vi "Intake Controller.vi"(8 "error in":errorcluster) -> ()   [LabVIEW 2019]
doc: "This VI executes continuously carrying out the current operation and responding to updates or new operations. It will often contain the timing or control code that is difficult to place directly in TeleOp. This VI generally opens all sensors and motors and isolates the rest of the robot code from knowing how the operations are carried out."
uses:
  <vilib>/Rock Robotics/WPI/Framework/Completion Status.ctl
  Intake Setpoints.ctl
  Intake Operations.ctl
  <vilib>/Rock Robotics/WPI/ThirdParty/Phoenix-LabVIEW/Motor Controller/Controls/CTRE_Phoenix_MotorControl_ControlMode.ctl
  <vilib>/Rock Robotics/Network Tables/NT Write Boolean.vi
panel:
  in  "Interactive Values":T1
  out "Current\nCmd":string
  in  "Buttons":cluster{"Execute Cmd":bool, "Abort Cmd":bool}
  out "Command Timing":cluster{"Start Time (ms)":u32, "Iterations":i32}
  out "Status":T3
  # "Tip: It may be helpful to observe inputs and sensor values.\nYou may also want to display tuning or debugging controls."
  # "Interactive Command: You may fill in the settings for a command\nand schedule it with the Execute button. You can observe and abort\nany command while fine tuning the code for the controller."
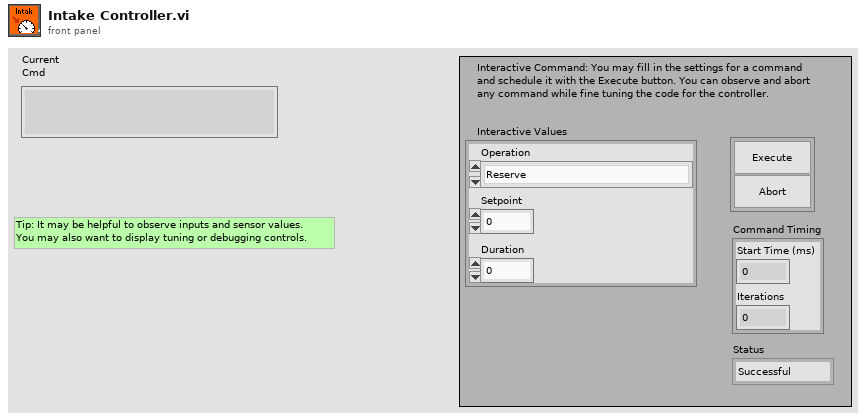
[diagram p1: front panel]
types:
  T1 = typedef "Intake Setpoints.ctl" = cluster{"Operation":T2, "Setpoint":dbl, "Duration":dbl}
  T2 = typedef "Intake Operations.ctl" = enum16{"Reserve", "Read Current", "Immediate", "Intake for time"}
  T3 = typedef "Completion Status.ctl" = enum16{"Successful", "Aborted", "Incomplete"}
  T4 = typedef "WPI_MotorControlDeviceRef.ctl" = cluster{"DeviceStatus":errorcluster, "Type":T5, "PWM":cluster{"PWM Channel":T6, "DeadBand":T7}, "CAN":cluster{"Device Number":u8, "SetOutput VI Ref":variant, "GetOutput VI Ref":variant, "Enable VI Ref":variant, "Disable VI Ref":variant, "Data":variant}, "Invert":bool, "DIO PWM":cluster{"PWM \"Enable\" Channel":T6, "DIOChannel":T8, "PWM Rate":dbl}}
  T5 = typedef "WPI_MotorControlType.ctl" = enum16{"PWM", "CAN", "DIO PWM"}
  T6 = typedef "FPGA_DIOPWMChannel.ctl" = enum8{"PWM 0", "PWM 1", "PWM 2", "PWM 3", "PWM 4", "PWM 5", "PWM 6", "PWM 7", "PWM 8", "PWM 9", "PWM MXP 0", "PWM MXP 1", "PWM MXP 2", "PWM MXP 3", "PWM MXP 4", "PWM MXP 5", "PWM MXP 6", "PWM MXP 7", "PWM MXP 8", "PWM MXP 9", "Invalid"}
  T7 = typedef "WPI_PWMDeadband.ctl" = cluster{"Name":string, "maxPositivePwm":i32, "minPositivePwm":i32, "centerPwm":i32, "maxNegativePwm":i32, "minNegativePwm":i32, "angularRange":u16}
  T8 = typedef "FPGA_DIOChannel.ctl" = enum8{"DIO 0", "DIO 1", "DIO 2", "DIO 3", "DIO 4", "DIO 5", "DIO 6", "DIO 7", "DIO 8", "DIO 9", "DIO MXP 0", "DIO MXP 1", "DIO MXP 2", "DIO MXP 3", "DIO MXP 4", "DIO MXP 5", "DIO MXP 6", "DIO MXP 7", "DIO MXP 8", "DIO MXP 9", "DIO MXP 10", "DIO MXP 11", "DIO MXP 12", "DIO MXP 13", "DIO MXP 14", "DIO MXP 15", "SPI Port CS1", "SPI Port CS2", "SPI Port CS3", "SPI Port MISO", "SPI Port MOSI", "Invalid"}
  T9 = typedef "Command Status Info.ctl" = cluster{"Name":string, "Status":T3, "notifier out":T10}
  T10 = typedef "Completion Notifier.ctl" = refnum<notifier>
  T11 = cluster{"Current Command":T1, "Command Timing":cluster{"Start Time (ms)":u32, "Iterations":i32}, "Command Arguments":cluster{"Command Info":T9, "Description":string, "Default Command":T1, "queue out":refnum<queue>, "Subsystem Name":string}}
  T12 = typedef "CTRE_Phoenix_MotorControl_ControlMode.ctl" = u16
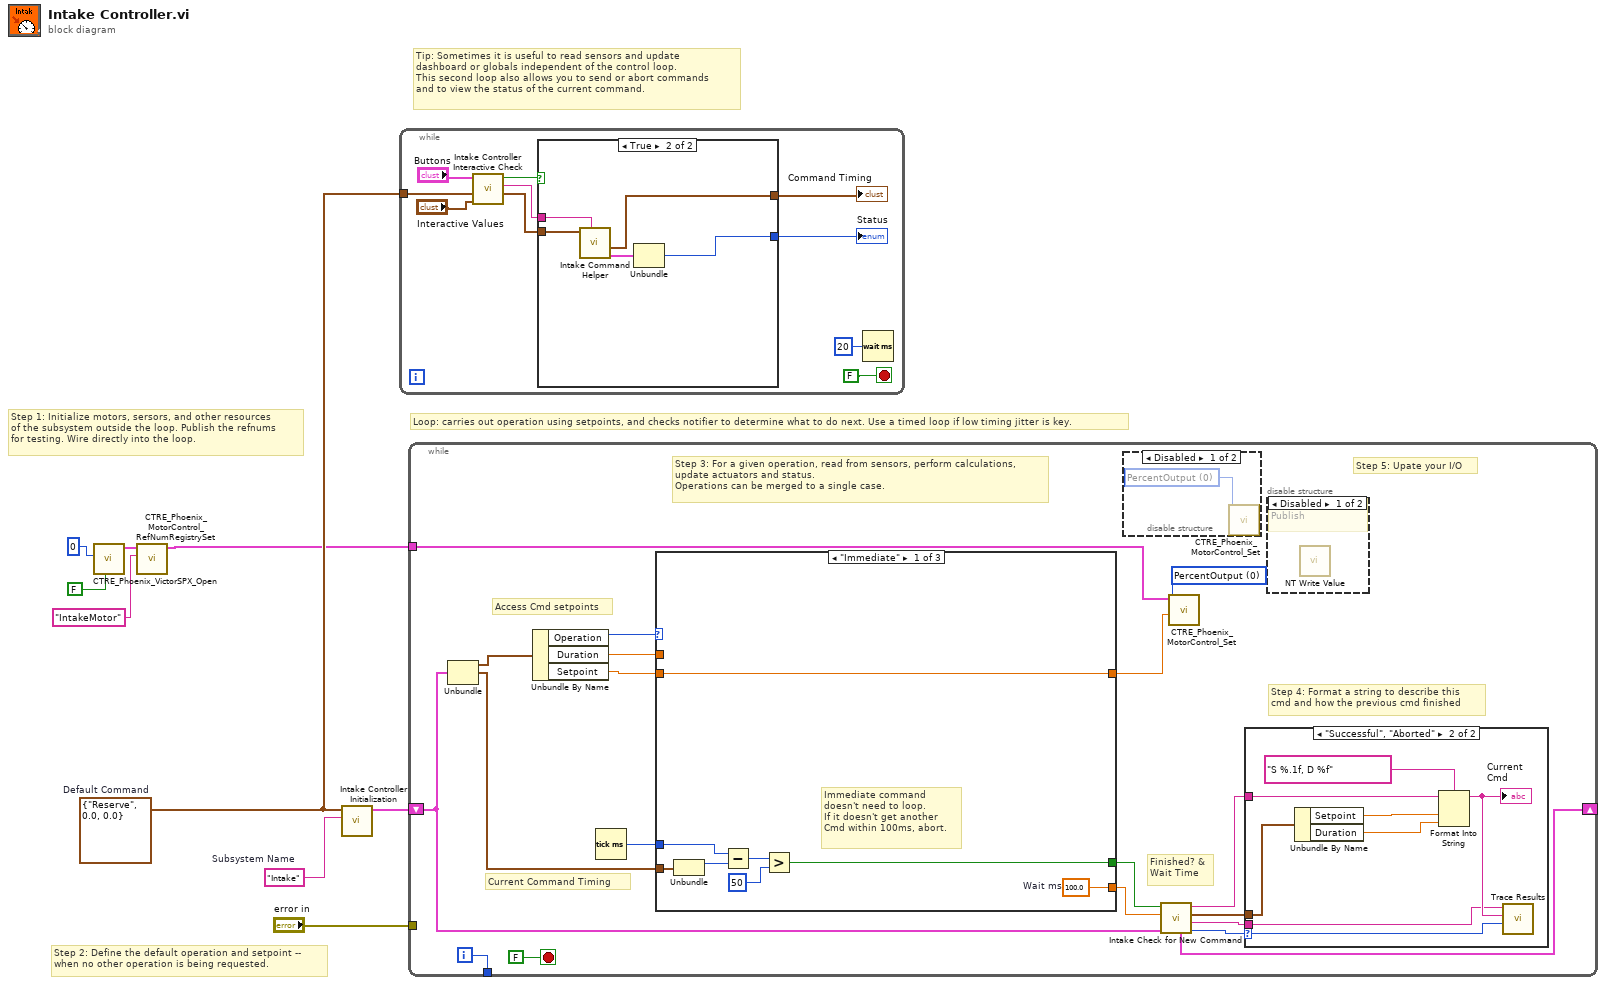
[diagram p0: block diagram]
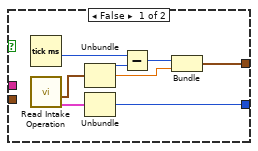
[diagram p2: hidden frame]
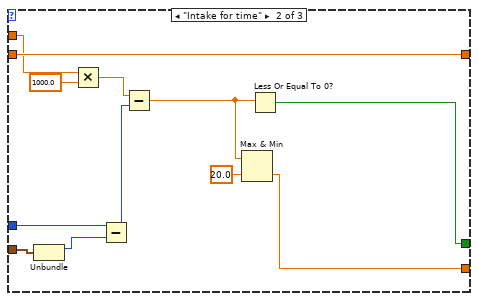
[diagram p6: hidden frame]
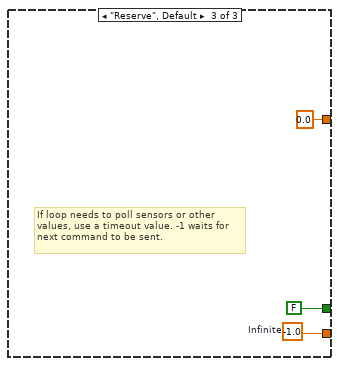
[diagram p7: hidden frame]
diagram:
  w6 = T1 {"Operation"=enum."Reserve", "Setpoint"=0.0, "Duration"=0.0}  # Default Command
  w7 = "Intake"  # Subsystem Name
  # "Tip: Sometimes it is useful to read sensors and update\ndashboard or globals independent of the control loop.\nThis second loop also allows you to send or abort commands\nand to view the status of the current command."
  # "Step 2: Define the default operation and setpoint --\nwhen no other operation is being requested."
  # "Step 1: Initialize motors, sersors, and other resources\nof the subsystem outside the loop. Publish the refnums\nfor testing. Wire directly into the loop."
  # "Loop: carries out operation using setpoints, and checks notifier to determine what to do next. Use a timed loop if low timing jitter is key."
  n1 = call <vilib>:"CTRE_Phoenix_VictorSPX_Open.vi"("Invert"=FALSE, "Device Number"=u8 0) -> ("CAN Talon SRX Ref"=w4:T4)  [unwired: 8 in, 1 out]
  n2 = call <vilib>:"CTRE_Phoenix_MotorControl_RefNumRegistrySet.vi"("refnum name"="IntakeMotor", "PhoenixMotorControlDevRef"=w4) -> ("PhoenixMotorControlDevRef"=w1:T4)  [unwired: 8 in, 1 out]
  n3 = call "Intake Controller Initialization.vi"("Subsystem Name"=w7, "Default Command"=w6) -> ("Current Command"=w8:T11)  [unwired: 9 in]
  n4 = while {
    tunnel: w6 -> [w16]
    stop <- FALSE stop-if-true
    n5 = call "Intake Controller Interactive Check.vi"("Interactive Command in"="Interactive Values", "Default Command"=w16, "Buttons"="Buttons") -> ("Interactive Command out"=w13:T1, "Trace String"=w14:string, "Schedule"=w15:bool)  [unwired: 6 in]
    n6 = case shown="True" w15 {
      tunnel: [w27 w32] -> w12
      tunnel: w13 -> [_ w30]
      tunnel: [w23 w28] -> w11
      tunnel: w14 -> [_ w31]
      frame False {
        n7 = Tick Count (ms)() -> (millisecond timer value=w22:u32)
        n8 = call "Read Intake Operation.vi"() -> ("Command Info"=w20:T9, "SubSystem Data"=w21:T1)  [unwired: 9 in, 1 out]
        n9 = Unbundle(w21) -> ("Operation"=w26:T2, "Setpoint"=w24:dbl)  [unwired: 1 out]
        n10 = Unbundle(w20) -> ("Status"=w27:T3)  [unwired: 2 out]
        n11 = Subtract(x=w22, y=w26) -> (x-y=w25:u32)
        n12 = Bundle(w25, "Setpoint"=w24) -> (w23:cluster{u32, "Setpoint":dbl})  [unwired: 1 in]
      }
      frame True {
        n13 = call "Intake Command Helper.vi"("Description"=w31, "SubSystem Data"=w30) -> ("Command Info Out"=w29:T9, "Command Timing"=w28:cluster{"Start Time (ms)":u32, "Iterations":i32})  [unwired: 7 in, 1 out]
        n14 = Unbundle(w29) -> ("Status"=w32:T3)  [unwired: 2 out]
      }
    }
    "Status" <- w12
    "Command Timing" <- w11
    n15 = Wait (ms)(milliseconds to wait=u32 20) -> ()  [unwired: 1 out]
  }
  n16 = while {
    shift-right: [w43] -> _
    shift-left: w8 -> [w36]
    tunnel: [w50] -> _
    tunnel: "error in" -> [_]
    tunnel: w1 -> [w33]
    i -> [w50]
    stop <- FALSE stop-if-true
    w35 = T12 0 items=["PercentOutput"=0, "Position"=1, "Velocity"=2, "Current"=3, "Follower"=5, "MotionProfile"=6, "MotionMagic"=7, "MotionProfileArc"=10, "Disabled"=15] ("Control Mode")
    # "Step 5: Upate your I/O"
    # "Step 4: Format a string to describe this\ncmd and how the previous cmd finished"
    # "Current Command Timing"
    # "Access Cmd setpoints"
    # "Finished? &\nWait Time"
    # "Step 3: For a given operation, read from sensors, perform calculations,\nupdate actuators and status.\nOperations can be merged to a single case."
    n17 = Unbundle(w36) -> ("Current Command"=w49:T1, "Command Timing"=w45:cluster{"Start Time (ms)":u32, "Iterations":i32})  [unwired: 1 out]
    n18 = Unbundle By Name(w49) -> ("Operation"=w48:T2, "Duration"=w47:dbl, "Setpoint"=w44:dbl)
    n19 = Tick Count (ms)() -> (millisecond timer value=w46:u32)
    n20 = case shown="\"Immediate\"" w48 {
      tunnel: [w68 w69 w83] -> w41
      tunnel: [w62 w72 FALSE ("ignore previous (F)")] -> w42
      tunnel: w45 -> [w64 w80 _]
      tunnel: w47 -> [_ w76 _]
      tunnel: w46 -> [w63 w78 _]
      tunnel: w44 -> [w61 w77 _]
      tunnel: [w61 w77 0.0 ("Setpoint")] -> w34
      frame "Immediate" {
        w68 = 100.0  # Wait ms
        # "Immediate command\ndoesn't need to loop.\nIf it doesn't get another\nCmd within 100ms, abort."
        n21 = Unbundle(w64) -> ("Start Time (ms)"=w67:u32)  [unwired: 1 out]
        n22 = Subtract(x=w63, y=w67) -> (x-y=w66:u32)
        n23 = Greater?(x=w66, y=u8 50 ("Left Motor")) -> (0:w62:bool)
      }
      frame "Intake for time" {
        n24 = Unbundle(w80) -> ("Start Time (ms)"=w79:u32)  [unwired: 1 out]
        n25 = Multiply(x=w76, y=1000.0) -> (x*y=w74:dbl)
        n26 = Subtract(x=w78, y=w79) -> (x-y=w73:u32)
        n27 = Subtract(x=w74, y=w73) -> (x-y=w70:dbl)
        n28 = Max & Min(x=w70, y=20.0) -> (min(x,y)=w69:dbl)  [unwired: 1 out]
        n29 = Less Or Equal To 0?(x=w70) -> (x <= 0?=w72:bool)
      }
      frame "Reserve", Default {
        w83 = -1.0  # Infinite
        # "If loop needs to poll sensors or other\nvalues, use a timeout value. -1 waits for\nnext command to be sent."
      }
    }
    n30 = disable-structure shown="Disabled" {
      frame Disabled {
        w52 = T12 0 items=["PercentOutput"=0, "Position"=1, "Velocity"=2, "Current"=3, "Follower"=5, "MotionProfile"=6, "MotionMagic"=7, "MotionProfileArc"=10, "Disabled"=15] ("Control Mode")
        n31 = call <vilib>:"CTRE_Phoenix_MotorControl_Set.vi"("Control Mode"=w52) -> ()  [unwired: 9 in, 2 out]
      }
      frame Enabled {
      }
    }
    n32 = call "Intake Check for New Command.vi"("Current Command"=w36, "Wait time (ms)"=w41, "Finished?"=w42) -> ("Completion"=w37:T3, "Subsystem Name"=w38:string, "Current Command"=w39:T1, "Initial Trace String"=w40:string, "NextCommand"=w43:T11)  [unwired: 4 in]
    n33 = call <vilib>:"CTRE_Phoenix_MotorControl_Set.vi"("Output"=w34, "Control Mode"=w35, "PhoenixMotorControlDevRef"=w33) -> ()  [unwired: 7 in, 2 out]
    n34 = case shown="\"Successful\", \"Aborted\"" w37 {
      selector: w37 -> [_ w60]
      tunnel: w40 -> [_ w56]
      tunnel: w39 -> [_ w57]
      tunnel: w38 -> [_ w53]
      frame "Incomplete", Default {
        # "Continuing current command"
      }
      frame "Successful", "Aborted" {
        # "Report and setup for next command"
        n35 = Unbundle By Name(w57) -> ("Setpoint"=w59:dbl, "Duration"=w54:dbl)
        n36 = Format Into String(format string="S %.1f, D %f", initial string=w56, w59, w54) -> (resulting string=w55:string)  [unwired: 1 in, 1 out]
        "Current\nCmd" <- w55
        n37 = call <vilib>:"Trace Results.vi"("Status of previous command"=w60, "Description"=w55, "Subsystem"=w53) -> ()  [unwired: 9 in]
      }
    }
    n38 = disable-structure shown="Disabled" {
      frame Disabled {
        # "Publish"
        n39 = call-poly <vilib>:"NT Write Value.vi"() -> ()  [unwired: 11 in, 1 out]
      }
      frame Enabled {
      }
    }
  }
